vi "Event Active.vi"(8 "error in (no error)":errorcluster, 11 "[MV] Key Certify in":refnum<class "[MV] Key Certify.lvclass">) -> (0 "error out":errorcluster, 3 "[MV] Key Certify out":refnum<class "[MV] Key Certify.lvclass">)   [LabVIEW 2023, in "[MV] Key Certify.lvlib" / "[MV] Key Certify.lvclass"]
uses:
  [MV] Key Certify.lvclass
  [MV] Key Certify.lvclass/[MV] Key Certify.ctl
  <vilib>/YU/YU_Encrypt/Base64/Base64.lvclass
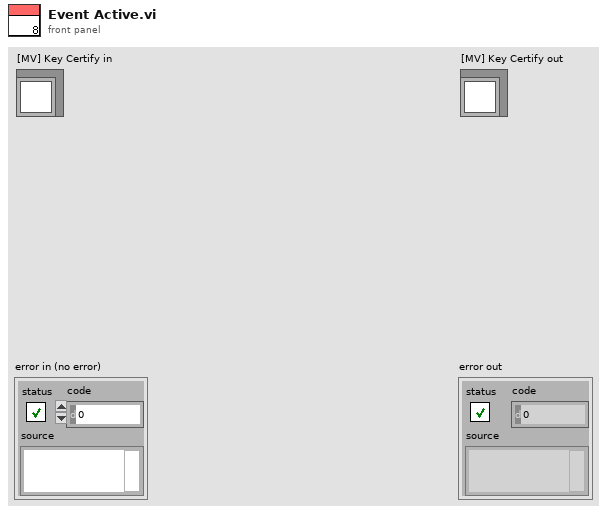
[diagram p1: front panel]
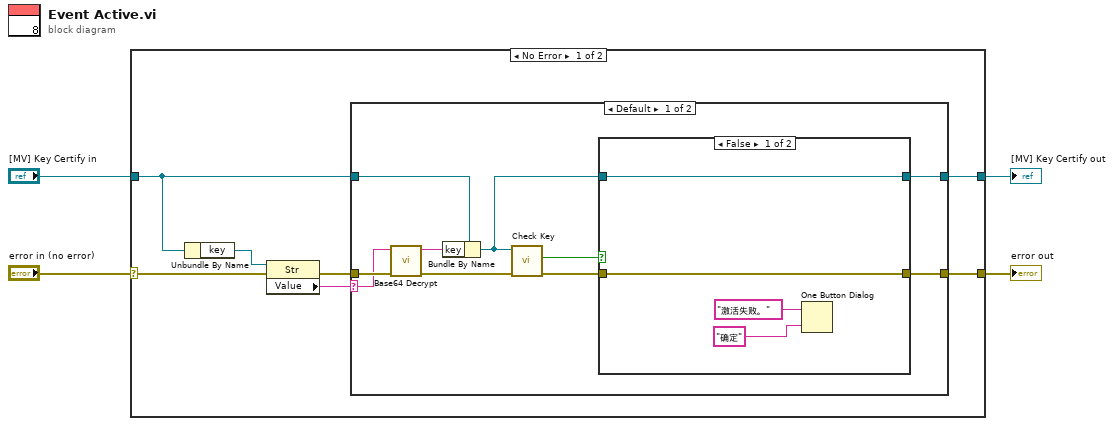
[diagram p0: block diagram]
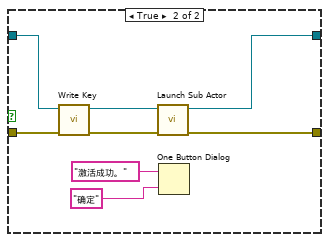
[diagram p2: hidden frame]
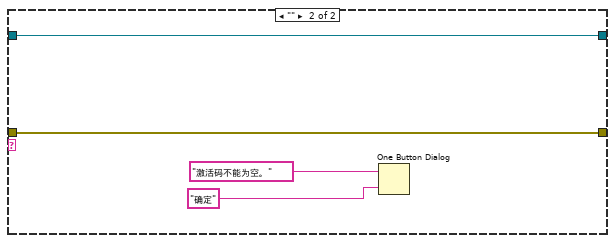
[diagram p3: hidden frame]
diagram:
  n1 = case shown="No Error" "error in (no error)" {
    selector: "error in (no error)" -> [w11 w39]
    tunnel: [w7 w39] -> w3
    tunnel: [w5 w38] -> w1
    tunnel: "[MV] Key Certify in" -> [w6 w38]
    frame No Error {
      n2 = Unbundle By Name(w6) -> ("key"=w10:refnum<vi>)
      n3 = property class="Str"(reference=w10, error in=w11) -> (error out=w9:errorcluster, "Value"=w8:string)  [unwired: 1 out]
      n4 = case shown="Default" w8 {
        selector: w8 -> [w12 _]
        tunnel: w9 -> [w15 w37]
        tunnel: [w17 w37] -> w7
        tunnel: w6 -> [w20 w34]
        tunnel: [w19 w34] -> w5
        frame Default {
          n5 = call <vilib>:"Base64 Decrypt.vi"("error in (no error)"=w15, "message_encrypted"=w12) -> ("error out"=w14:errorcluster, "message"=w13:string)  [unwired: 8 in]
          n6 = Bundle By Name(cluster=w20, "key"=w13) -> (w16:refnum<class "[MV] Key Certify.lvclass">)
          n7 = call "Check Key.vi"("error in (no error)"=w14, "[MV] Key Certify in"=w16) -> ("error out"=w18:errorcluster, "valid?"=w21:bool)  [unwired: 7 in, 1 out]
          n8 = case shown="False" w21 {
            tunnel: w16 -> [w25 w30]
            tunnel: [w25 w27] -> w19
            tunnel: w18 -> [w24 w31]
            tunnel: [w24 w26] -> w17
            frame False {
              n9 = One Button Dialog(message="激活失败。", button name ("OK")="确定") -> ()  [unwired: 1 out]
            }
            frame True {
              n10 = call "Write Key.vi"("error in (no error)"=w31, "[MV] Key Certify in"=w30) -> ("error out"=w28:errorcluster, "[MV] Key Certify out"=w29:refnum<class "[MV] Key Certify.lvclass">)  [unwired: 8 in]
              n11 = call "Launch Sub Actor.vi"("error in (no error)"=w28, "[MV] Key Certify in"=w29) -> ("error out"=w26:errorcluster, "[MV] Key Certify out"=w27:refnum<class "[MV] Key Certify.lvclass">)  [unwired: 8 in]
              n12 = One Button Dialog(message="激活成功。", button name ("OK")="确定") -> ()  [unwired: 1 out]
            }
          }
        }
        frame "" {
          n13 = One Button Dialog(message="激活码不能为空。", button name ("OK")="确定") -> ()  [unwired: 1 out]
        }
      }
    }
    frame Error {
    }
  }
  "error out" <- w3
  "[MV] Key Certify out" <- w1
